vi "ServiceChannels.GetRefs.vi"(8 "error in (no error)":errorcluster, 11 "Item Ref in":T1 format="%.0x") -> (0 "error out":errorcluster, 1 "Status":T1[](array[typedef]) format="%.0x", 2 "Trigger":T1[](array[typedef]) format="%.0x", 3 "Section Ref out":T1 format="%.0x")   [LabVIEW 2019, in "Diagnostics Addon System Explorer.lvlib"]
uses:
  Diagnostics Addon System Explorer.lvlib
  <vilib>/NI VeriStand/Custom Device API/Custom Device Item Ref.ctl
  Addon Shared/SubVIs/Constants.vi
  <vilib>/NI VeriStand/Custom Device Tools/Custom Device Utility Library/NI VeriStand - Search for Item by GUID.vi
  <vilib>/NI VeriStand/Custom Device Tools/Custom Device Utility Library/NI VeriStand - Search for Item by Name.vi
  <vilib>/NI VeriStand/Custom Device Tools/Custom Device Utility Library/Custom Device Utility Library.lvlib
  Addon Shared/Diagnostics Addon Shared.lvlib
  <vilib>/NI VeriStand/Custom Device API/Custom Device API.lvlib
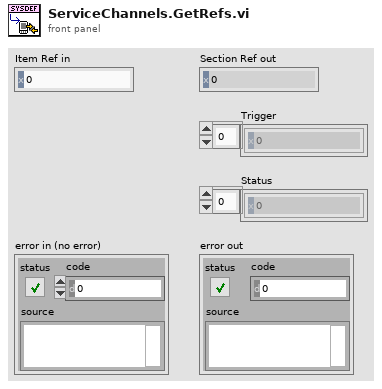
[diagram p1: front panel]
types:
  T1 = typedef "Custom Device API.lvlib/Custom Device Item Ref.ctl" = u64
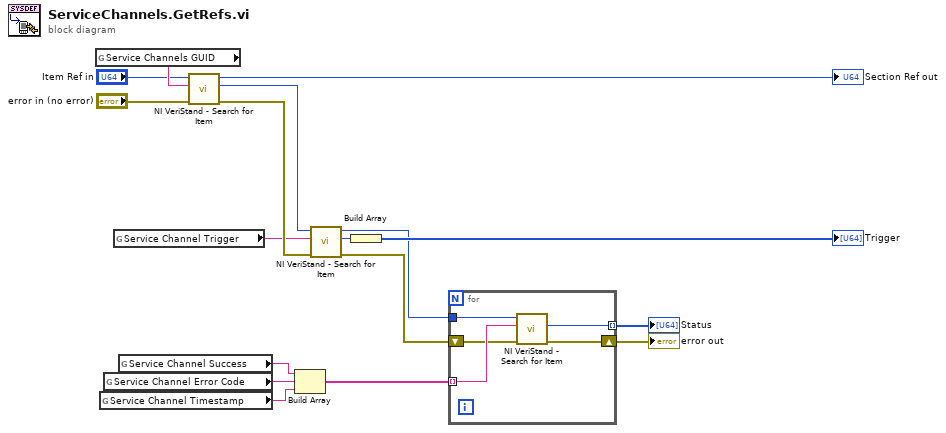
[diagram p0: block diagram]
diagram:
  n1 = global read "Constants.vi" "Service Channels GUID"() -> (w7:string)
  n2 = global read "Constants.vi" "Service Channel Timestamp"() -> (w11:string)
  n3 = global read "Constants.vi" "Service Channel Error Code"() -> (w10:string)
  n4 = global read "Constants.vi" "Service Channel Trigger"() -> (w9:string)
  n5 = global read "Constants.vi" "Service Channel Success"() -> (w3:string)
  n6 = call-poly <vilib>:"NI VeriStand - Search for Item.vi"("error in"="error in (no error)", "Item GUID"=w7, "Section Ref in"="Item Ref in") -> ("error out"=w15:errorcluster, "Item Ref"=w8:T1, "Section Ref out"=→"Section Ref out":T1)  [unwired: 5 in, 1 out]
  n7 = Build Array(w3, w10, w11) -> (w12:string[])
  n8 = call-poly <vilib>:"NI VeriStand - Search for Item.vi"("error in"=w15, "Item Name"=w9, "Section Ref in"=w8) -> ("error out"=w1:errorcluster, "Item Ref"=w13:T1, "Section Ref out"=w2:T1)  [unwired: 5 in, 1 out]
  n9 = Build Array(w13) -> (→"Trigger":T1[])
  n10 = for {
    tunnel: w12 -> [w22] mode=indexing
    shift-right: [w20] -> w16
    shift-left: w1 -> [w21]
    tunnel: w2 -> [w19]
    tunnel: [w18] -> w14 mode=indexing
    n11 = call-poly <vilib>:"NI VeriStand - Search for Item.vi"("error in"=w21, "Item Name"=w22, "Section Ref in"=w19) -> ("error out"=w20:errorcluster, "Item Ref"=w18:T1)  [unwired: 5 in, 2 out]
  }
  "error out" <- w16
  "Status" <- w14
